vi "create.vi"(8 "error in":errorcluster) -> (0 "error out":errorcluster, 3 "queue reporter out":refnum<class "queue reporter.lvclass">)   [LabVIEW 2013, in "queue reporter.lvclass"]
uses:
  queue reporter.lvclass
  result/result.lvclass
  queue reporter.lvclass/queue reporter.ctl
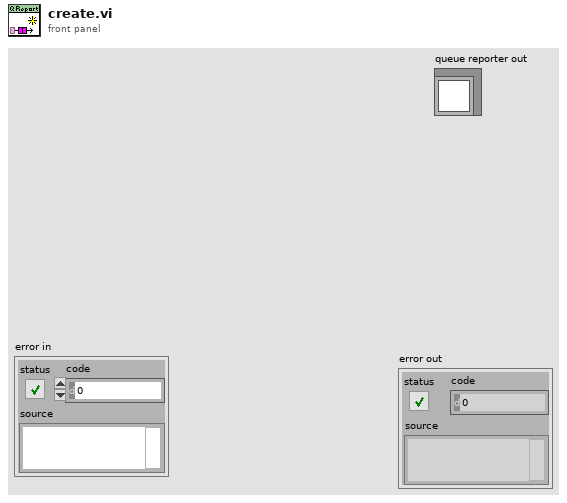
[diagram p1: front panel]
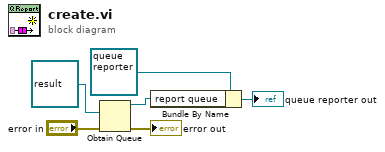
[diagram p0: block diagram]
diagram:
  n1 = Obtain Queue(element data type=refnum<class "result.lvclass"> refnum ("result"), error in (no error)="error in") -> (queue out=w1:refnum<queue>, error out=→"error out":errorcluster)  [unwired: 3 in, 1 out]
  n2 = Bundle By Name(cluster=refnum<class "queue reporter.lvclass"> refnum ("queue reporter in"), "report queue"=w1) -> (→"queue reporter out":refnum<class "queue reporter.lvclass">)
